vi "ex3.vi"() -> ()   [LabVIEW 2022 SP3]
panel:
  in  "Array":bool[](array[boolean])
  out "data":string
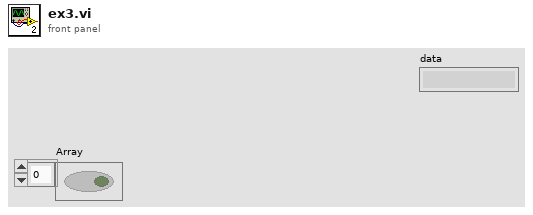
[diagram p1: front panel]
types:
  T1 = enum16{"open", "replace", "create", "open or create", "replace or create", "replace or create with confirmation"}
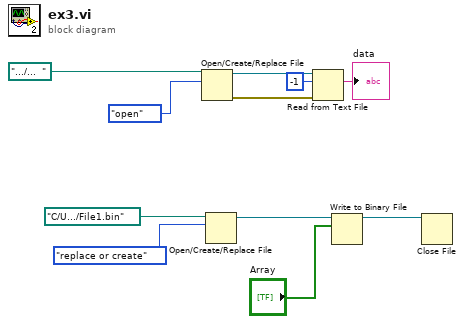
[diagram p0: block diagram]
diagram:
  n1 = Open/Create/Replace File(file path (use dialog)=path ".../...  ", operation (0:open)=T1."open") -> (refnum out=w9:refnum<file>, error out=w7:errorcluster)  [unwired: 4 in, 1 out]
  n2 = Open/Create/Replace File(file path (use dialog)=path "C:/U.../File1.bin", operation (0:open)=T1."replace or create") -> (refnum out=w3:refnum<file>)  [unwired: 4 in, 2 out]
  n3 = Read from Text File(file (use dialog)=w9, count=-1, error in=w7) -> (text=→"data":string)  [unwired: 1 in, 3 out]
  n4 = Write to Binary File(file (use dialog)=w3, data="Array") -> (refnum out=w1:refnum<file>)  [unwired: 4 in, 2 out]
  n5 = Close File(refnum=w1) -> ()  [unwired: 1 in, 2 out]
